vi "Nephelometer.vi"(8 "error in":errorcluster) -> (0 "error out":errorcluster)   [LabVIEW 2015]
uses:
  Reusable/Session APIs/File Access/Config Data/Config Session.ctl
  Reusable/Session APIs/File Access/Config Data/Config Data.lvclass
  Devices/Nephelometer/Neph File Observer/Neph File Obs.lvclass
  Devices/Nephelometer/Nephelometer.lvclass
  Reusable/Session Log/System Log.lvclass
  Reusable/Session APIs/Serial/Serial Session.lvclass
  Reusable/Session APIs/Text Communication/Text Device Session.lvclass
  <vilib>/Platform/TimedLoop/XDataNode/timing_clust.ctl
  <vilib>/Platform/TimedLoop/XDataNode/nitl_modes.ctl
  <vilib>/Platform/TimedLoop/XDataNode/wakeup.ctl
  Reusable/Session Log/System Log.lvclass/System Log.ctl
  Reusable/Session APIs/File Access/Config Data/Config Data.lvclass/Config Data.ctl
  Devices/Configurable Device/Configurable Device.lvclass/Configurable Device.ctl
  Reusable/File IO/Class/File Observer.lvclass/File Observer.ctl
  Devices/Nephelometer/Nephelometer.lvclass/Nephelometer.ctl
  Reusable/Session APIs/Text Communication/Text Device Session.lvclass/Text Device Session.ctl
  Reusable/Session Log/Accessors/Write Main Path.vi
  Reusable/Session APIs/File Access/Config Data/Accessors/Read Ref.vi
  Reusable/File IO/Class/Accessors/Write Top Data Path.vi
  Reusable/File IO/Class/Accessors/Write File Prefix.vi
  Reusable/File IO/Class/Accessors/Write File Ext.vi
  Reusable/File IO/Class/Accessors/Write File Header.vi
  Reusable/File IO/Class/Accessors/Write Max Size.vi
  Reusable/File IO/Class/Write SwitchonDate_.vi
  Reusable/File IO/Class/Write SwitchonSize_.vi
  Devices/Configurable Device/Write Handle.vi
  Reusable/Session APIs/Text Communication/Write hSysLog.vi
  Devices/Nephelometer/Accessors/Write Session Handle.vi
  <vilib>/Utility/config.llb/Read Key (Path).vi
  Devices/Nephelometer/Unpolled Commands/Set Autozero Time.vi
  Devices/Nephelometer/Unpolled Commands/Set Autozero Period.vi
  <userlib>/_Session Fwk/Session - Root.lvclass
  <vilib>/Platform/TimedLoop/XDataNode/XDataNode.xnode
  <vilib>/Platform/TimedLoop/XDataNode/XDNodeRunTimeDep.lvlib
  <vilib>/Utility/config.llb/NI_LVConfig.lvlib
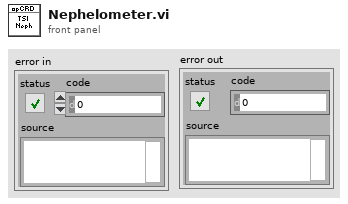
[diagram p1: front panel]
types:
  T1 = typedef "Config Data.lvclass/Config Session.ctl" = refnum<data-value>
  T2 = typedef "Session - Root.lvclass/Session Handle.ctl" = refnum<data-value>
  T3 = typedef "NI_LVConfig.lvlib/Config Data RefNum.ctl" = refnum<k1>
  T4 = typedef "XDNodeRunTimeDep.lvlib/timing_clust.ctl" = cluster{"Expected End [f-1]":u64, "Actual End [f-1]":u64, "Finished Late? [f-1]":bool, "Expected End [i-1]":u64, "Actual End [i-1]":u64, "Finished Late? [i-1]":bool, "Expected Start [i]":u64, "Actual Start [i]":u64, "Expected Start [f]":u64, "Actual Start [f]":u64, "Source Name":string, "Structure Name":string, "Period":i64, "Deadline":i64, "Offset":i64, "Start":i64, "Priority":i32, "Timeout":i32, "Mode":T5, "Wakeup Reason":T6, "Error":errorcluster, "Source Type":string, "Secondary Source Type":string, "Global End Time":u64, "Global Start Time":u64, "Frame Duration":u64, "Iteration Duration":u64, "Assigned CPU":i32, "I/O Scan Engine Mode":u32}
  T5 = typedef "XDNodeRunTimeDep.lvlib/nitl_modes.ctl" = enum32{"No Change", "Process missed periods, maintain original phase", "Discard missed periods, maintain original phase", "Process missed periods, ignore original phase", "Discard missed periods, ignore original phase"}
  T6 = typedef "XDNodeRunTimeDep.lvlib/wakeup.ctl" = enum32{"Normal", "Aborted", "Asynchronous wakeup", "Timing source error", "Timed loop error", "Timeout"}
  T7 = cluster{"Sensitivity":dbl, "Pressure":dbl, "Tsample":dbl, "Tinlet":dbl, "RH":dbl, "Vlamp":dbl, "Ilamp":dbl}
  T8 = cluster{"Mode":enum16{"Normal", "Zero", "Blank"}, "Scatter Mode":enum16{"Total Scatter", "Back Scatter"}, "Time in Mode":i32, "Cblue":dbl, "Cgreen":dbl, "Cred":dbl, "Cback,blue":dbl, "Cback,green":dbl, "Cback,red":dbl}
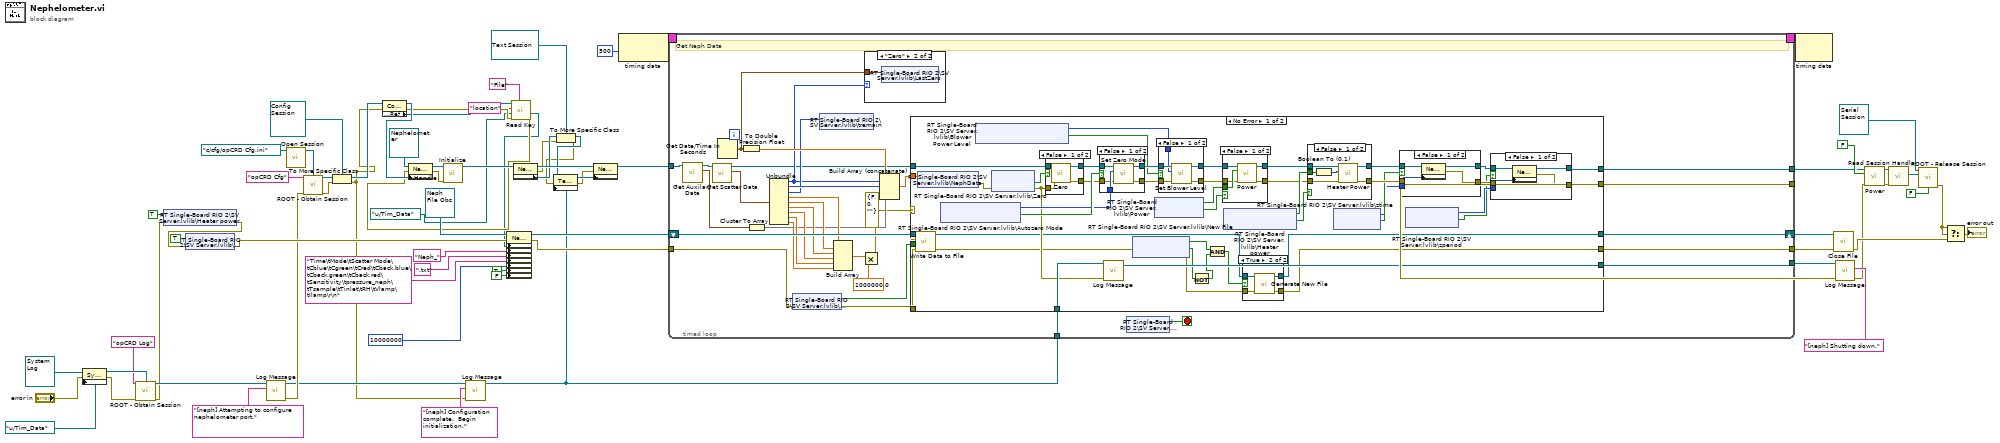
[diagram p0: block diagram]
diagram:
  n1 = property class="Sys Log"(reference=refnum<class "System Log.lvclass"> refnum ("Sys Log"), error in="error in", "Accessors:Main Path"=path "u:/Tim_Data" ("RD Data Path")) -> (reference out=w28:refnum<class "System Log.lvclass">, error out=w27:errorcluster)
  n2 = call <userlib>:"ROOT - Obtain Session.vi"("Session Name ()"="opCRD Log", "OBJ - Session"=w28, "error in (no error)"=w27) -> ("Session Handle"=w25:T2, "error out"=w23:errorcluster)  [unwired: 10 in, 1 out]
  n3 = shared-variable "RT Single-Board RIO 2\\SV Server.lvlib\\Heater power"(TRUE ("Heater power"), error in=w23) -> (error out=w67:errorcluster)
  n4 = shared-variable "RT Single-Board RIO 2\\SV Server.lvlib\\Power"(TRUE ("Blower Pwr"), error in=w67) -> (error out=w66:errorcluster)
  n5 = call "Log Message.vi"("MSG In"="[neph] Attempting to configure nephelometer port.", "session in"=w25) -> ("error out"=w43:errorcluster, "session out"=w42:T2)  [unwired: 8 in]
  n6 = call "Open Session.vi"("Path"=path "c:/cfg/opCRD Cfg.ini") -> ("Config Data"=w48:refnum<class "Config Data.lvclass">)  [unwired: 9 in, 1 out]
  n7 = call <userlib>:"ROOT - Obtain Session.vi"("Session Name ()"="opCRD Cfg", "OBJ - Session"=w48, "error in (no error)"=w43) -> ("Session Handle"=w51:T2, "error out"=w52:errorcluster)  [unwired: 10 in, 1 out]
  n8 = To More Specific Class(target class=T1 refnum ("Session Handle"), reference=w51, error in=w52) -> (specific class reference=w22:T1, error out=w21:errorcluster)
  n9 = property class="Config Data"(reference=w22, error in=w21) -> (reference out=w20:T1, error out=w18:errorcluster, "Accessors:Ref"=w19:T3)
  n10 = call "Log Message.vi"("error in"=w21, "MSG In"="[neph] Configuration complete.  Begin initialization.", "session in"=w42) -> ("session out"=w40:T2)  [unwired: 7 in, 1 out]
  n11 = call-poly <vilib>:"Read Key.vi"("section"="File", "error in (no error)"=w18, "default value"=path "u:/Tim_Data" ("RD Data Path"), "key"="location", "refnum"=w19) -> ("error out"=w17:errorcluster, "value"=w13:path)  [unwired: 3 in, 2 out]
  n12 = property class="Neph"(reference=refnum<class "Nephelometer.lvclass"> refnum ("Neph"), error in=w17, "Accessors:Handle"=w20) -> (reference out=w53:refnum<class "Nephelometer.lvclass">, error out=w54:errorcluster)
  n13 = call "Initialize.vi"("error in"=w54, "Neph In"=w53) -> ("Neph Out"=w56:refnum<class "Nephelometer.lvclass">)  [unwired: 8 in, 1 out]
  n14 = property class="Neph File Obs"(reference=refnum<class "Neph File Obs.lvclass"> refnum ("Neph File Obs"), error in=w66, "Data Access:Top Data Path"=w13, "Data Access:File Prefix"="Neph_" ("File Prefix"), "Data Access:File Ext"=".txt" ("File Ext"), "Data Access:File Header"="Time\tMode\tScatter Mode\tCblue\tCgreen\tCred\tCback,blue\tCback,green\tCback,red\tSensitivity\tpressure_neph\tTsample\tTinlet\tRH\tVlamp\tIlamp\r\n" ("File Header"), "Data Access:Max Size"=i64 10000000 ("Max Size"), "Accessors:SwitchonDate_"=TRUE ("SwitchonDate_"), "Accessors:SwitchonSize_"=FALSE ("SwitchonSize_")) -> (reference out=w60:refnum<class "Neph File Obs.lvclass">, error out=w61:errorcluster)
  n15 = property class="Neph"(reference=w56) -> (reference out=w39:refnum<class "Nephelometer.lvclass">, error out=w5:errorcluster, "Accessors:Session Handle"=w8:T2)  [unwired: 1 in]
  n16 = To More Specific Class(target class=refnum<data-value> refnum ("Session Handle"), reference=w8, error in=w5) -> (specific class reference=w6:refnum<data-value>, error out=w4:errorcluster)
  n17 = property class="Text Session"(reference=w6, error in=w4, "Accessors:hSysLog"=w40) -> (reference out=w38:refnum<data-value>, error out=w31:errorcluster)
  n18 = property class="Neph"(reference=w39, error in=w31, "Accessors:Session Handle"=w38) -> (reference out=w37:refnum<class "Nephelometer.lvclass">)  [unwired: 1 out]
  n19 = node-c288(i64 500 ("Period")) -> (w74:T4)
  n20 = timed-loop {
    tunnel: w37 -> [w80]
    tunnel: [w105] -> w69
    timing: w74 -> [_]
    timing-out: [_] -> w73
    tunnel: w61 -> [w86]
    tunnel: [w84] -> w63
    shift-right: [w87] -> w62
    shift-left: w60 -> [w104]
    tunnel: [w100] -> w34
    tunnel: w40 -> [w99]
    tunnel: [w98] -> w36
    stop <- w101 stop-if-true
    # "Get Neph Data"
    n21 = call "Get Auxilary Data.vi"("Neph in"=w80) -> ("Auxilary data"=w77:T7, "Neph out"=w79:refnum<class "Nephelometer.lvclass">)  [unwired: 8 in, 1 out]
    n22 = call "Get Scatter Data.vi"("Neph in"=w79) -> ("Data Record"=w78:T8, "Neph out"=w76:refnum<class "Nephelometer.lvclass">)  [unwired: 8 in, 1 out]
    n23 = Get Date/Time In Seconds() -> (seconds since 1Jan1904=w81:timestamp)
    n24 = To Double Precision Float(number=w81) -> (double precision float=w106:dbl)
    n25 = Cluster To Array(cluster=w77) -> (array=w88:dbl[])
    n26 = Unbundle(w78) -> ("Mode"=w82:enum16{"Normal", "Zero", "Blank"}, "Scatter Mode"=w107:enum16{"Total Scatter", "Back Scatter"}, "Time in Mode"=w83:i32, "Cblue"=w97:dbl, "Cgreen"=w96:dbl, "Cred"=w95:dbl, "Cback,blue"=w94:dbl, "Cback,green"=w93:dbl, "Cback,red"=w92:dbl)
    n27 = shared-variable "RT Single-Board RIO 2\\SV Server.lvlib\\Write?"(error in=w86) -> (w102:bool, error out=w85:errorcluster)
    n28 = shared-variable "RT Single-Board RIO 2\\SV Server.lvlib\\tremain"(w83) -> ()  [unwired: 1 in, 1 out]
    n29 = Build Array(w97, w96, w95, w94, w93, w92) -> (w91:dbl[])
    n30 = Multiply(x=w91, y=1000000.0 ("Cback,red")) -> (x*y=w89:dbl[])
    n31 = case shown="\"Zero\"" w82 {
      tunnel: w81 -> [_ w108]
      frame "Normal", Default {
      }
      frame "Zero" {
        n32 = shared-variable "RT Single-Board RIO 2\\SV Server.lvlib\\LastZero"(w108) -> ()  [unwired: 1 in, 1 out]
      }
    }
    n33 = Build Array (concatenate)(w106, w82, w107, w89, w88) -> (w103:dbl[])
    n34 = case shown="No Error" errorcluster {"status"=FALSE, "code"=0, "source"=""} ("error IO") {
      selector: errorcluster {"status"=FALSE, "code"=0, "source"=""} ("error IO") -> [_ w207]
      tunnel: w76 -> [w153 w211]
      tunnel: [w109 w211] -> w105
      tunnel: w104 -> [w139 w210]
      tunnel: w103 -> [w138 _]
      tunnel: w102 -> [w137 _]
      tunnel: [w110 w207] -> w100
      tunnel: w99 -> [w131 w208]
      tunnel: [w129 w208] -> w98
      tunnel: [w126 w210] -> w87
      tunnel: w85 -> [w124 w209]
      tunnel: [w123 w209] -> w84
      frame No Error {
        n35 = call "Write Data to File.vi"("error in"=w124, "Write?"=w137, "Data In"=w138, "Neph File Obs in"=w139) -> ("error out"=w125:errorcluster, "Neph File Obs out"=w127:refnum<class "Neph File Obs.lvclass">)  [unwired: 6 in]
        n36 = shared-variable "RT Single-Board RIO 2\\SV Server.lvlib\\NephData"(w138) -> (error out=w136:errorcluster)  [unwired: 1 in]
        n37 = shared-variable "RT Single-Board RIO 2\\SV Server.lvlib\\Autozero Mode"() -> (w149:u8, w151:bool)  [unwired: 2 in, 1 out]
        n38 = shared-variable "RT Single-Board RIO 2\\SV Server.lvlib\\Blower Power Level"() -> (w146:u8, w147:bool)  [unwired: 2 in, 1 out]
        n39 = shared-variable "RT Single-Board RIO 2\\SV Server.lvlib\\Zero"(error in=w136) -> (error out=w130:errorcluster, w152:bool)  [unwired: 1 in, 1 out]
        n40 = case shown="False" w152 {
          tunnel: w153 -> [w204 w206]
          tunnel: [w203 w206] -> w150
          tunnel: w130 -> [w202 w205]
          tunnel: [w201 w205] -> w135
          frame False {
            n41 = call "Zero.vi"("error in"=w202, "Neph in"=w204) -> ("error out"=w201:errorcluster, "Neph out"=w203:refnum<class "Nephelometer.lvclass">)  [unwired: 8 in]
          }
          frame True {
          }
        }
        n42 = case shown="False" w151 {
          tunnel: w150 -> [w198 w200]
          tunnel: [w197 w200] -> w148
          tunnel: w149 -> [w196 _]
          tunnel: w135 -> [w195 w199]
          tunnel: [w194 w199] -> w134
          frame False {
            n43 = call "Set Zero Mode.vi"("error in"=w195, "Mode"=w196, "Neph in"=w198) -> ("error out"=w194:errorcluster, "Neph out"=w197:refnum<class "Nephelometer.lvclass">)  [unwired: 7 in]
          }
          frame True {
          }
        }
        n44 = call "Log Message.vi"("error in"=w130, "session in"=w131) -> ("session out"=w129:T2)  [unwired: 8 in, 1 out]
        n45 = shared-variable "RT Single-Board RIO 2\\SV Server.lvlib\\New File"(error in=w125) -> (w120:bool, error out=w128:errorcluster, w122:bool)  [unwired: 1 in]
        n46 = shared-variable "RT Single-Board RIO 2\\SV Server.lvlib\\Power"() -> (w144:bool, w143:bool)  [unwired: 2 in, 1 out]
        n47 = case shown="False" w147 {
          tunnel: w148 -> [w191 w193]
          tunnel: [w190 w193] -> w145
          tunnel: w146 -> [w189 _]
          tunnel: w134 -> [w188 w192]
          tunnel: [w187 w192] -> w133
          frame False {
            n48 = call "Set Blower Level.vi"("error in"=w188, "Level"=w189, "Neph in"=w191) -> ("error out"=w187:errorcluster, "Neph out"=w190:refnum<class "Nephelometer.lvclass">)  [unwired: 7 in]
          }
          frame True {
          }
        }
        n49 = Not(x=w122) -> (.not. x?=w121:bool)
        n50 = And(x=w120, y=w121) -> (x .and. y?=w119:bool)
        n51 = case shown="False" w143 {
          tunnel: w145 -> [w184 w186]
          tunnel: [w183 w186] -> w142
          tunnel: w144 -> [w182 _]
          tunnel: w133 -> [w181 w185]
          tunnel: [w180 w185] -> w132
          frame False {
            n52 = call "Power.vi"("error in"=w181, "Power?"=w182, "Neph in"=w184) -> ("error out"=w180:errorcluster, "Neph out"=w183:refnum<class "Nephelometer.lvclass">)  [unwired: 7 in]
          }
          frame True {
          }
        }
        n53 = shared-variable "RT Single-Board RIO 2\\SV Server.lvlib\\Heater power"() -> (w140:bool, w141:bool)  [unwired: 2 in, 1 out]
        n54 = case shown="True" w119 {
          tunnel: w128 -> [w167 w171]
          tunnel: [w166 w170] -> w126
          tunnel: [w167 w169] -> w123
          tunnel: w127 -> [w166 w168]
          frame False {
          }
          frame True {
            n55 = call-dynamic "Generate New File.vi"("error in"=w171, "File Obs in"=w168) -> ("error out"=w169:errorcluster, "File Obs out"=w170:refnum<class "Neph File Obs.lvclass">)  [unwired: 7 in, 1 out]
          }
        }
        n56 = case shown="False" w141 {
          tunnel: w142 -> [w177 w179]
          tunnel: [w176 w179] -> w118
          tunnel: w140 -> [w175 _]
          tunnel: w132 -> [w173 w178]
          tunnel: [w172 w178] -> w117
          frame False {
            n57 = Boolean To (0,1)(Boolean=w175) -> (0, 1=w174:i16)
            n58 = call "Heater Power.vi"("error in"=w173, "On/Off"=w174, "Neph in"=w177) -> ("error out"=w172:errorcluster, "Neph out"=w176:refnum<class "Nephelometer.lvclass">)  [unwired: 7 in]
          }
          frame True {
          }
        }
        n59 = shared-variable "RT Single-Board RIO 2\\SV Server.lvlib\\ztime"() -> (w115:u16, w116:bool)  [unwired: 2 in, 1 out]
        n60 = case shown="False" w116 {
          tunnel: w118 -> [w163 w165]
          tunnel: [w162 w165] -> w114
          tunnel: [w161 w164] -> w113
          tunnel: w117 -> [_ w164]
          tunnel: w115 -> [w160 _]
          frame False {
            n61 = property class="Neph"(reference=w163, "Commands:Autozero Time"=w160) -> (reference out=w162:refnum<class "Nephelometer.lvclass">, error out=w161:errorcluster)  [unwired: 1 in]
          }
          frame True {
          }
        }
        n62 = shared-variable "RT Single-Board RIO 2\\SV Server.lvlib\\zperiod"() -> (w112:u16, w111:bool)  [unwired: 2 in, 1 out]
        n63 = case shown="False" w111 {
          tunnel: w114 -> [w157 w159]
          tunnel: [w156 w159] -> w109
          tunnel: [w155 w158] -> w110
          tunnel: w113 -> [_ w158]
          tunnel: w112 -> [w154 _]
          frame False {
            n64 = property class="Neph"(reference=w157, "Commands:Autozero Period"=w154) -> (reference out=w156:refnum<class "Nephelometer.lvclass">, error out=w155:errorcluster)  [unwired: 1 in]
          }
          frame True {
          }
        }
      }
      frame Error {
      }
    }
    n65 = shared-variable "RT Single-Board RIO 2\\SV Server.lvlib\\Stop"() -> (w101:bool)  [unwired: 1 in, 1 out]
  }
  n66 = node-c288(w73) -> ()  [unwired: 1 out]
  n67 = call-dynamic "Close File.vi"("error in"=w63, "File Obs in"=w62) -> ("error out"=w46:errorcluster)  [unwired: 8 in, 1 out]
  n68 = call "Log Message.vi"("error in"=w34, "MSG In"="[neph] Shutting down.", "session in"=w36) -> ("error out"=w33:errorcluster)  [unwired: 7 in, 1 out]
  n69 = call "Power.vi"("error in"=w33, "Power?"=FALSE, "Neph in"=w69) -> ("error out"=w47:errorcluster, "Neph out"=w70:refnum<class "Nephelometer.lvclass">)  [unwired: 7 in]
  n70 = call "Read Session Handle.vi"("error in (no error)"=w47, "Nephelometer in"=w70) -> ("Session Handle"=w11:T2)  [unwired: 7 in, 2 out]
  n71 = call <userlib>:"ROOT - Release Session.vi"("OBJ - Session in"=refnum<class "Serial Session.lvclass"> refnum ("Serial Session"), "Session Handle in"=w11, "force destroy? (F)"=FALSE) -> ("error out"=w9:errorcluster)  [unwired: 11 in, 1 out]
  n72 = Select(t=w9, s=w9, f=w46) -> (s? t:f=→"error out":errorcluster)
